vi "LINC COSMOS Append Array Item.vi"(5 "ignore":bool, 8 "error in (no error)":errorcluster, 9 "packet fields":T2, 10 "packet index":i32, 11 "packets in":T3[](array[typedef])) -> (0 "error out":errorcluster, 2 "item index":i32, 3 "packets out":T3[](array[typedef]))   [LabVIEW 2018, in "STEPkgDriver_LINC.lvlib"]
uses:
  STEPkgDriver_LINC.lvlib
  LINC Format Prototype.ctl
  LINC Packet.ctl
  LINC Packet Fields.ctl
  LINC Macro.ctl
panel:
  in  "macro":T1
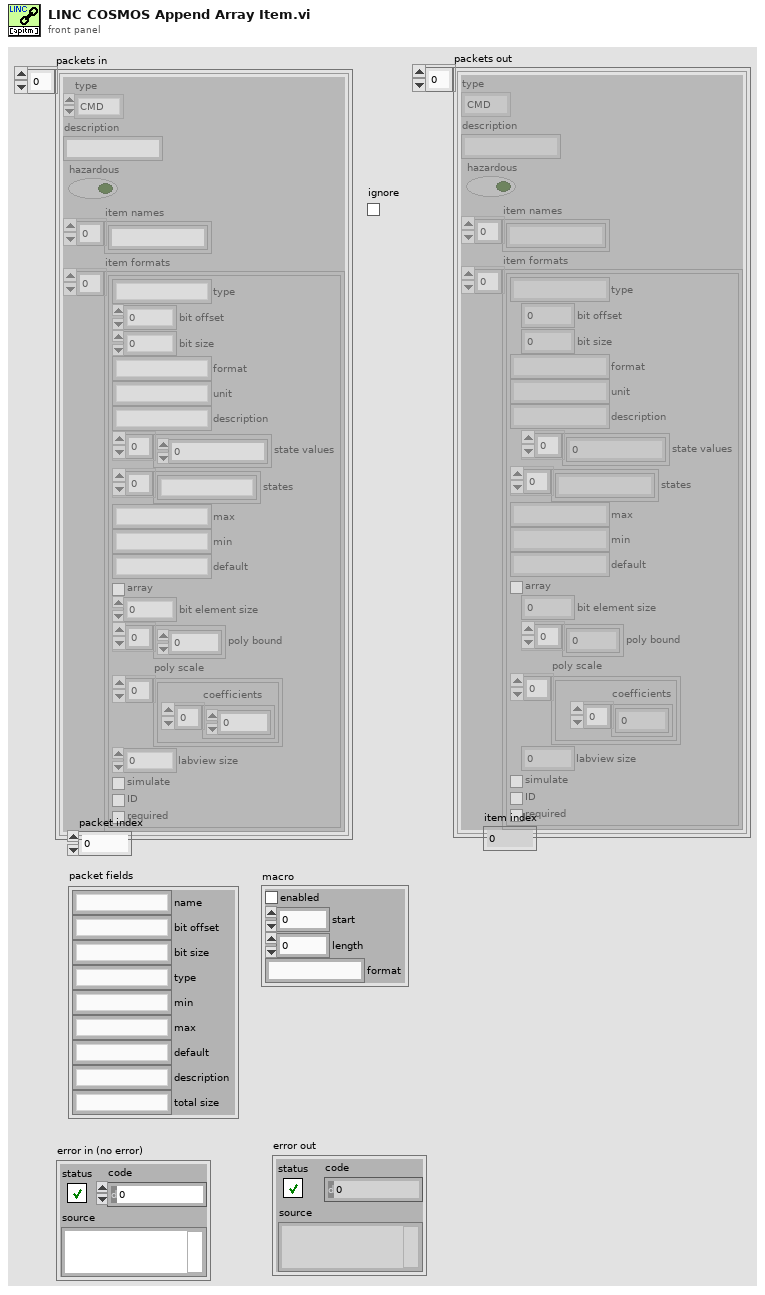
[diagram p1: front panel]
types:
  T1 = typedef "STEPkgDriver_LINC.lvlib/LINC Macro.ctl" = cluster{"enabled":bool, "start":i32, "length":i32, "format":string}
  T2 = typedef "STEPkgDriver_LINC.lvlib/LINC Packet Fields.ctl" = cluster{"name":string, "bit offset":string, "bit size":string, "type":string, "min":string, "max":string, "default":string, "description":string, "total size":string}
  T3 = typedef "STEPkgDriver_LINC.lvlib/LINC Packet.ctl" = cluster{"type":enum16{"CMD", "TLM"}, "description":string, "hazardous":bool, "item names":string[], "item formats":T4[]}
  T4 = typedef "STEPkgDriver_LINC.lvlib/LINC Format Prototype.ctl" = cluster{"type":string, "bit offset":i32, "bit size":i32, "format":string, "unit":string, "description":string, "state values":i64[], "states":string[], "max":string, "min":string, "default":string, "array":bool, "bit element size":i32, "poly bound":dbl[], "poly scale":cluster{"coefficients":dbl[]}[], "labview size":i32, "simulate":bool, "ID":bool, "required":bool}
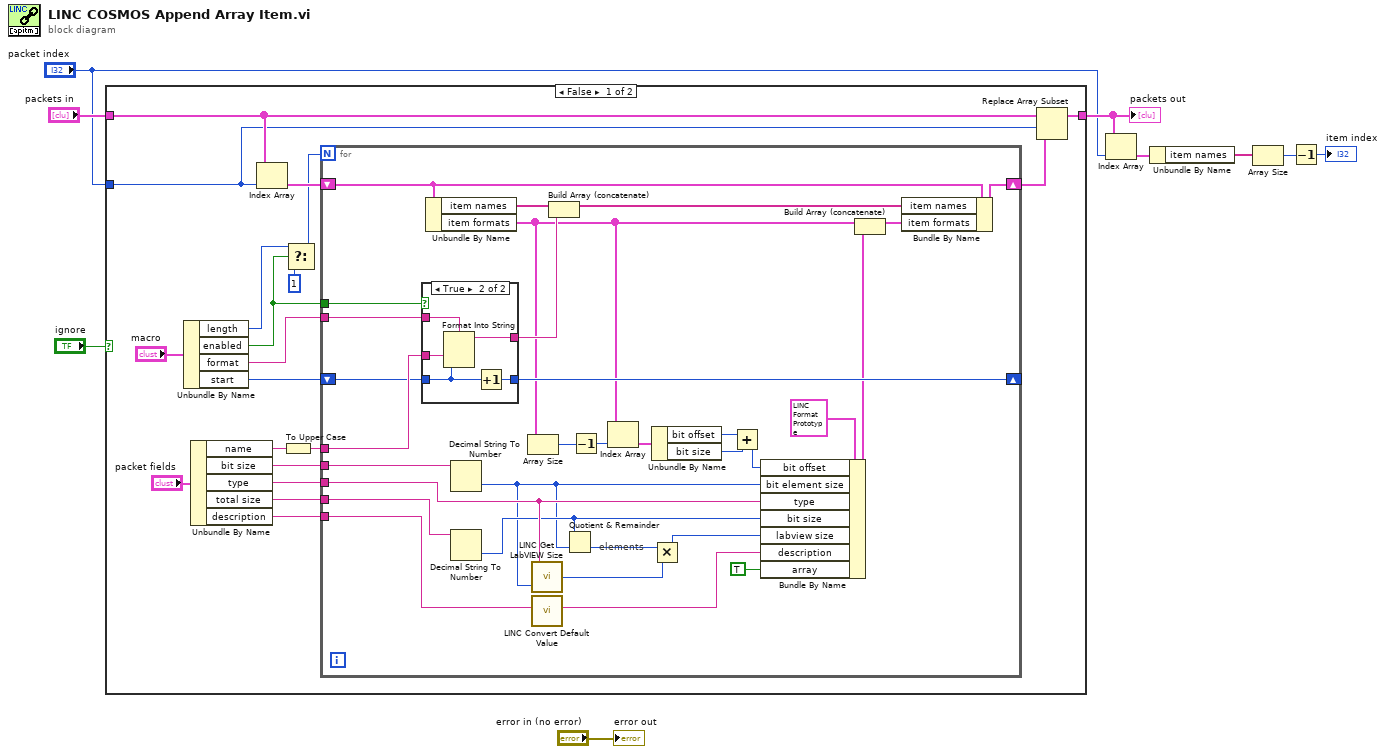
[diagram p0: block diagram]
diagram:
  n1 = case shown="False" "ignore" {
    tunnel: "packets in" -> [w13 w67]
    tunnel: [w12 w67] -> w3
    tunnel: "packet index" -> [w11 _]
    frame False {
      n2 = Unbundle By Name("macro") -> ("length"=w15:i32, "enabled"=w16:bool, "format"=w14:string, "start"=w19:i32)
      n3 = Unbundle By Name("packet fields") -> ("name"=w27:string, "bit size"=w26:string, "type"=w25:string, "total size"=w24:string, "description"=w23:string)
      n4 = Index Array(array=w13, index=w11) -> (element=w21:T3)
      n5 = To Upper Case(1:w27) -> (0:w28:string)
      n6 = Select(t=w15, s=w16, f=1) -> (s? t:f=w17:i32)
      n7 = for {
        N: w17 -> [_]
        tunnel: w28 -> [w55]
        tunnel: w26 -> [w37]
        tunnel: w25 -> [w36]
        tunnel: w24 -> [w35]
        tunnel: w23 -> [w34]
        shift-right: [w56] -> w20
        shift-left: w21 -> [w57]
        shift-right: [w53] -> _
        shift-left: w19 -> [w54]
        tunnel: w14 -> [w52]
        tunnel: w16 -> [w51]
        # "elements"
        n8 = case shown="True" w51 {
          tunnel: w55 -> [w61 w64]
          tunnel: [w61 w66] -> w50
          tunnel: w52 -> [_ w65]
          tunnel: w54 -> [w60 w63]
          tunnel: [w60 w62] -> w53
          frame False {
          }
          frame True {
            n9 = Format Into String(format string=w65, w64, w63) -> (resulting string=w66:string)  [unwired: 2 in, 1 out]
            n10 = Increment(x=w63) -> (x+1=w62:i32)
          }
        }
        n11 = Unbundle By Name(w57) -> ("item names"=w59:string[], "item formats"=w43:T4[])
        n12 = Decimal String To Number(string=w37) -> (number=w32:i32)  [unwired: 2 in, 1 out]
        n13 = Decimal String To Number(string=w35) -> (number=w33:i32)  [unwired: 2 in, 1 out]
        n14 = Array Size(array=w43) -> (size(s)=w49:i32)
        n15 = call "LINC Get LabVIEW Size.vi"("bit size"=w32, "type"=w36) -> ("labview size"=w30:i32)
        n16 = call "LINC Convert Default Value.vi"("default in"=w34) -> ("default out"=w41:string)  [unwired: 10 in]
        n17 = Build Array (concatenate)(w59, w50) -> (w58:string[])
        n18 = Quotient & Remainder(x=w33, y=w32) -> (floor(x/y)=w31:i32)  [unwired: 1 out]
        n19 = Decrement(x=w49) -> (x-1=w45:i32)
        n20 = Index Array(array=w43, index=w45) -> (element=w46:T4)
        n21 = Unbundle By Name(w46) -> ("bit offset"=w47:i32, "bit size"=w48:i32)
        n22 = Multiply(x=w31, y=w30) -> (x*y=w29:i32)
        n23 = Add(x=w47, y=w48) -> (x+y=w38:i32)
        n24 = Bundle By Name(cluster=T4 {"type"="", "bit offset"=0, "bit size"=0, "format"="", "unit"="", "description"="", "state values"=[], "states"=[], "max"="", "min"="", "default"="", "array"=FALSE, "bit element size"=0, "poly bound"=[], "poly scale"=[], "labview size"=0, "simulate"=FALSE, "ID"=FALSE, "required"=FALSE} ("data"), "bit offset"=w38, "bit element size"=w32, "type"=w36, "bit size"=w33, "labview size"=w29, "description"=w41, "array"=TRUE) -> (w39:T4)
        n25 = Build Array (concatenate)(w43, w39) -> (w44:T4[])
        n26 = Bundle By Name(cluster=w57, "item names"=w58, "item formats"=w44) -> (w56:T3)
      }
      n27 = Replace Array Subset(array=w13, new element=w20, index=w11) -> (w12:T3[])
    }
    frame True {
    }
  }
  "packets out" <- w3
  n28 = Index Array(array=w3, index="packet index") -> (element=w6:T3)
  n29 = Unbundle By Name(w6) -> ("item names"=w5:string[])
  n30 = Array Size(array=w5) -> (size(s)=w4:i32)
  n31 = Decrement(x=w4) -> (x-1=→"item index":i32)
  "error out" <- "error in (no error)"
